vi "Control_ReadJoystick.vi"(2 "Player":u8) -> (16 "Joystick":T1)   [LabVIEW 2018]
uses:
  TypDefs/Joystick_Enum.ctl
  <vilib>/Platform/TimedLoop/XDataNode/timing_clust.ctl
  <vilib>/Platform/TimedLoop/XDataNode/nitl_modes.ctl
  <vilib>/Platform/TimedLoop/XDataNode/wakeup.ctl
  <vilib>/rvi/Emulation/niFpgaSctlEmulationGetInTimedLoop.vi
  <vilib>/rvi/Emulation/niFpgaEmulationReportErrorSimple.vi
  <vilib>/rvi/Emulation/niFpgaGetClockAttributes.vi
  <vilib>/rvi/Emulation/niFpgaCriticalErrorInLSC.vi
  <vilib>/platform/TimedLoop/XDataNode/XDataNode.xnode
  <vilib>/Platform/TimedLoop/XDataNode/XDNodeRunTimeDep.lvlib
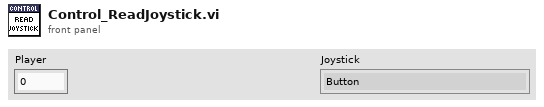
[diagram p1: front panel]
types:
  T1 = typedef "Joystick_Enum.ctl" = enum8{"Button", "Left", "Right", "Up", "Down", "None"}
  T2 = typedef "XDNodeRunTimeDep.lvlib/timing_clust.ctl" = cluster{"Expected End [f-1]":u64, "Actual End [f-1]":u64, "Finished Late? [f-1]":bool, "Expected End [i-1]":u64, "Actual End [i-1]":u64, "Finished Late? [i-1]":bool, "Expected Start [i]":u64, "Actual Start [i]":u64, "Expected Start [f]":u64, "Actual Start [f]":u64, "Source Name":string, "Structure Name":string, "Period":i64, "Deadline":i64, "Offset":i64, "Start":i64, "Priority":i32, "Timeout":i32, "Mode":T3, "Wakeup Reason":T4, "Error":errorcluster, "Source Type":string, "Secondary Source Type":string, "Global End Time":u64, "Global Start Time":u64, "Frame Duration":u64, "Iteration Duration":u64, "Assigned CPU":i32, "I/O Scan Engine Mode":u32}
  T3 = typedef "XDNodeRunTimeDep.lvlib/nitl_modes.ctl" = enum32{"No Change", "Process missed periods, maintain original phase", "Discard missed periods, maintain original phase", "Process missed periods, ignore original phase", "Discard missed periods, ignore original phase"}
  T4 = typedef "XDNodeRunTimeDep.lvlib/wakeup.ctl" = enum32{"Normal", "Aborted", "Asynchronous wakeup", "Timing source error", "Timed loop error", "Timeout"}
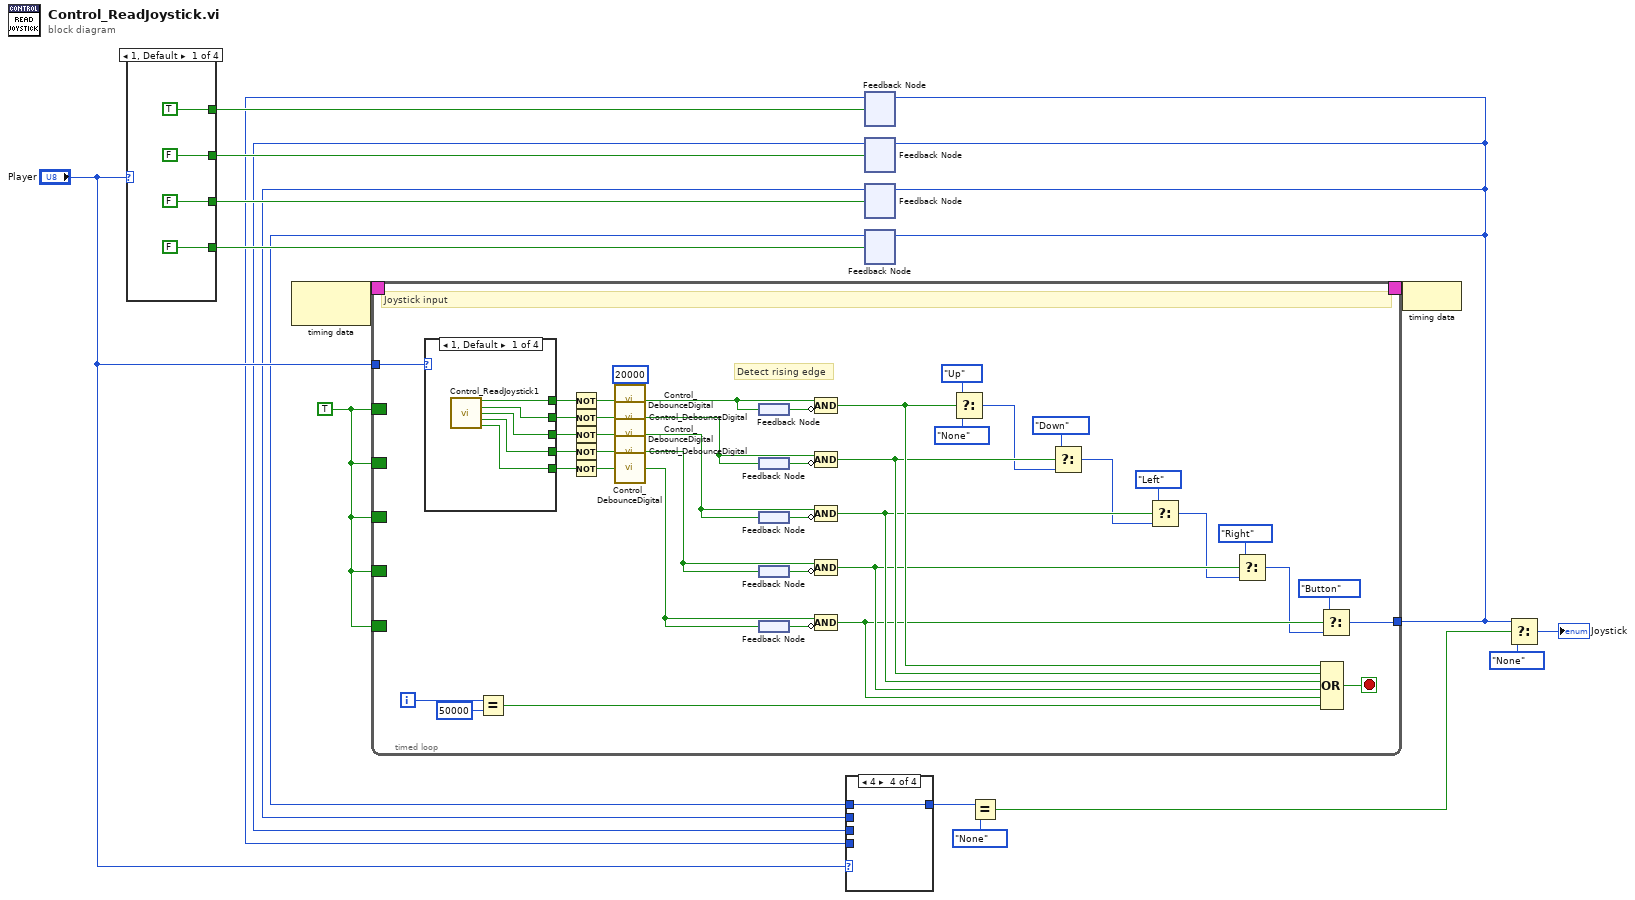
[diagram p0: block diagram]
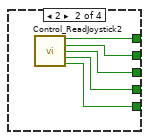
[diagram p5: hidden frame]
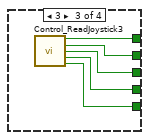
[diagram p6: hidden frame]
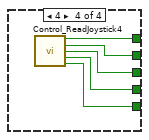
[diagram p7: hidden frame]
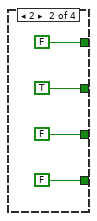
[diagram p8: hidden frame]
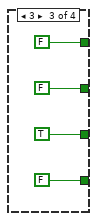
[diagram p9: hidden frame]
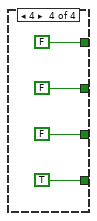
[diagram p10: hidden frame]
diagram:
  w15 = TRUE ("Output Filtered Signal")
  n1 = case shown="1, Default" "Player" {
    tunnel: [TRUE FALSE FALSE FALSE] -> w14
    tunnel: [FALSE TRUE FALSE FALSE] -> w13
    tunnel: [FALSE FALSE TRUE FALSE] -> w12
    tunnel: [FALSE FALSE FALSE TRUE] -> w11
    frame 1, Default {
    }
    frame 2 {
    }
    frame 3 {
    }
    frame 4 {
    }
  }
  n2 = node-c288() -> (w17:T2)  [unwired: 1 in]
  n3 = timed-loop {
    tunnel: [w55] -> w10
    timing: w17 -> [_]
    timing-out: [_] -> w16
    border: w15 -> [_]
    border: w15 -> [_]
    border: w15 -> [_]
    border: w15 -> [_]
    border: w15 -> [_]
    tunnel: "Player" -> [w35]
    i -> [w54]
    stop <- w71 stop-if-true
    w36 = u16 20000 ("Cycles to Filter")
    # "Detect rising edge"
    # "Joystick input"
    n4 = case shown="1, Default" w35 {
      tunnel: [w81 w86 w91 w96] -> w46
      tunnel: [w80 w85 w90 w95] -> w45
      tunnel: [w79 w84 w89 w94] -> w44
      tunnel: [w78 w83 w88 w93] -> w43
      tunnel: [w77 w82 w87 w92] -> w42
      frame 1, Default {
        n5 = call "Control_ReadJoystick1.vi"() -> ("Up"=w81:bool, "Down"=w80:bool, "Left"=w79:bool, "Right"=w78:bool, "Button"=w77:bool)  [unwired: 11 in]
      }
      frame 2 {
        n6 = call "Control_ReadJoystick2.vi"() -> ("Up"=w86:bool, "Down"=w85:bool, "Left"=w84:bool, "Right"=w83:bool, "Button"=w82:bool)  [unwired: 11 in]
      }
      frame 3 {
        n7 = call "Control_ReadJoystick3.vi"() -> ("Up"=w91:bool, "Down"=w90:bool, "Left"=w89:bool, "Right"=w88:bool, "Button"=w87:bool)  [unwired: 11 in]
      }
      frame 4 {
        n8 = call "Control_ReadJoystick4.vi"() -> ("Up"=w96:bool, "Down"=w95:bool, "Left"=w94:bool, "Right"=w93:bool, "Button"=w92:bool)  [unwired: 11 in]
      }
    }
    n9 = Equal?(x=w54, y=50000) -> (x = y?=w52:bool)
    n10 = Not(x=w46) -> (.not. x?=w51:bool)
    n11 = Not(x=w45) -> (.not. x?=w50:bool)
    n12 = Not(x=w44) -> (.not. x?=w49:bool)
    n13 = Not(x=w43) -> (.not. x?=w48:bool)
    n14 = Not(x=w42) -> (.not. x?=w47:bool)
    n15 = call "Control_DebounceDigital.vi"("Input Signal"=w51, "Cycles to Filter"=w36) -> ("Output Filtered Signal"=w76:bool)
    n16 = call "Control_DebounceDigital.vi"("Input Signal"=w50, "Cycles to Filter"=w36) -> ("Output Filtered Signal"=w75:bool)
    n17 = call "Control_DebounceDigital.vi"("Input Signal"=w49, "Cycles to Filter"=w36) -> ("Output Filtered Signal"=w74:bool)
    n18 = call "Control_DebounceDigital.vi"("Input Signal"=w48, "Cycles to Filter"=w36) -> ("Output Filtered Signal"=w73:bool)
    n19 = call "Control_DebounceDigital.vi"("Input Signal"=w47, "Cycles to Filter"=w36) -> ("Output Filtered Signal"=w72:bool)
    n20 = feedback #1() -> (w41:bool)
    n21 = feedback-in #1(w76) -> ()
    n22 = feedback #2() -> (w40:bool)
    n23 = feedback-in #2(w75) -> ()
    n24 = feedback #3() -> (w39:bool)
    n25 = feedback-in #3(w74) -> ()
    n26 = feedback #4() -> (w38:bool)
    n27 = feedback-in #4(w73) -> ()
    n28 = feedback #5() -> (w37:bool)
    n29 = feedback-in #5(w72) -> ()
    n30 = Compound Arithmetic op=AND(w76, invert w41) -> (w70:bool)
    n31 = Compound Arithmetic op=AND(w75, invert w40) -> (w67:bool)
    n32 = Compound Arithmetic op=AND(w74, invert w39) -> (w63:bool)
    n33 = Compound Arithmetic op=AND(w73, invert w38) -> (w60:bool)
    n34 = Compound Arithmetic op=AND(w72, invert w37) -> (w57:bool)
    n35 = Select(t=Joystick_Enum."Up" ("Joystick"), s=w70, f=Joystick_Enum."None") -> (s? t:f=w66:T1)
    n36 = Select(t=Joystick_Enum."Down" ("Joystick"), s=w67, f=w66) -> (s? t:f=w62:T1)
    n37 = Select(t=Joystick_Enum."Left" ("Joystick"), s=w63, f=w62) -> (s? t:f=w59:T1)
    n38 = Select(t=Joystick_Enum."Right" ("Joystick"), s=w60, f=w59) -> (s? t:f=w56:T1)
    n39 = Select(t=Joystick_Enum."Button" ("Joystick"), s=w57, f=w56) -> (s? t:f=w55:T1)
    n40 = Compound Arithmetic op=OR(w70, w67, w63, w60, w57, w52) -> (w71:bool)
  }
  n41 = feedback #6() -> (w9:T1)  [unwired: 1 in]
  n42 = feedback-in #6(w10, w14) -> ()
  n43 = feedback #7() -> (w6:T1)  [unwired: 1 in]
  n44 = feedback-in #7(w10, w13) -> ()
  n45 = feedback #8() -> (w5:T1)  [unwired: 1 in]
  n46 = feedback-in #8(w10, w12) -> ()
  n47 = feedback-in #9(w10, w11) -> ()
  n48 = feedback #9() -> (w4:T1)  [unwired: 1 in]
  n49 = case shown="4" "Player" {
    tunnel: w9 -> [w99 _ _ _]
    tunnel: w6 -> [_ w100 _ _]
    tunnel: w5 -> [_ _ w101 _]
    tunnel: w4 -> [_ _ _ w102]
    tunnel: [w99 w100 w101 w102] -> w1
    frame 1, Default {
    }
    frame 2 {
    }
    frame 3 {
    }
    frame 4 {
    }
  }
  n50 = Equal?(x=w1, y=Joystick_Enum."None") -> (x = y?=w2:bool)
  n51 = node-c288(w16) -> ()
  n52 = Select(t=w10, s=w2, f=Joystick_Enum."None") -> (s? t:f=→"Joystick":T1)
